vi "host run 2.vi"() -> ()   [LabVIEW 2012]
panel:
  out "Frame Rate":dbl
  out "Image":T1(plugin-control)
  in  "stop":bool
  out "Image 2":T1(plugin-control)
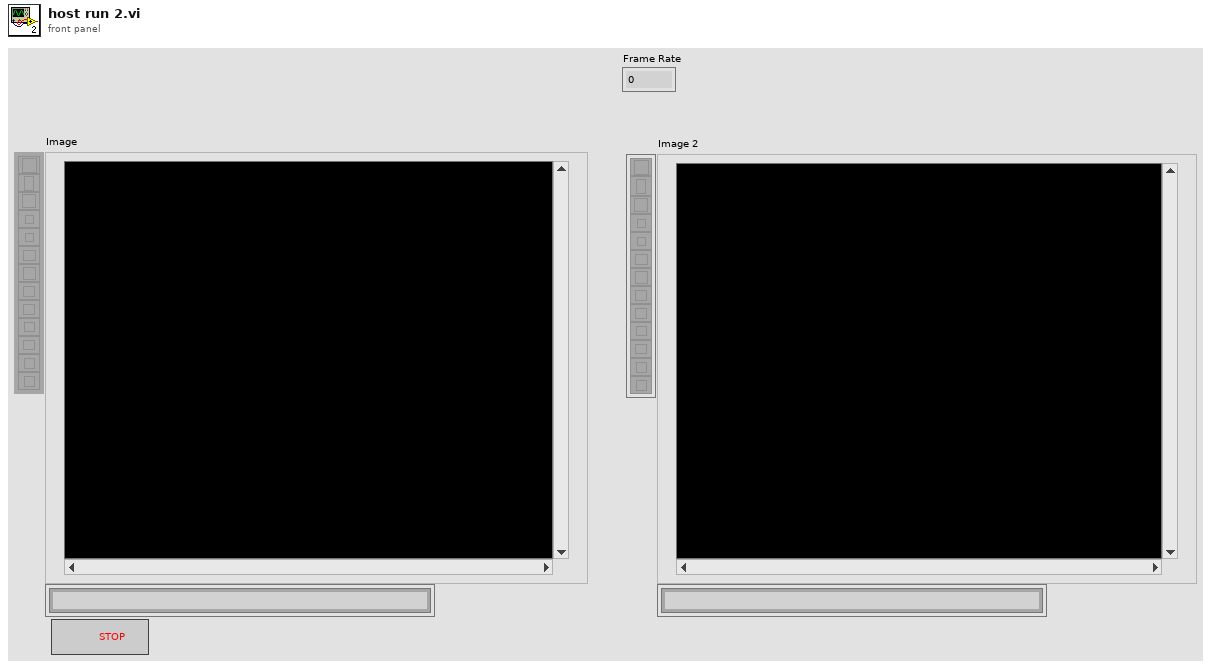
[diagram p1: front panel]
types:
  T1 = typedef "IMAQ Image.ctl" = refnum<image>
  T2 = cluster{"Global Rectangle":cluster{"x1Left":i32, "y1Top":i32, "x2Right":i32, "y2Bottom":i32}, "Centroid":cluster{"x":sgl, "y":sgl}, "Object Size":u32, "Score":dbl}[]
  T3 = cluster{"Shape Report (Shape Matching 1)[0]":cluster{"Global Rectangle":cluster{"x1Left":i32, "y1Top":i32, "x2Right":i32, "y2Bottom":i32}, "Centroid":cluster{"x":sgl, "y":sgl}, "Object Size":u32, "Score":dbl}, "Shape Report (Shape Matching 1)[1]":cluster{"Global Rectangle":cluster{"x1Left":i32, "y1Top":i32, "x2Right":i32, "y2Bottom":i32}, "Centroid":cluster{"x":sgl, "y":sgl}, "Object Size":u32, "Score":dbl}, "Shape Report (Shape Matching 1)[2]":cluster{"Global Rectangle":cluster{"x1Left":i32, "y1Top":i32, "x2Right":i32, "y2Bottom":i32}, "Centroid":cluster{"x":sgl, "y":sgl}, "Object Size":u32, "Score":dbl}, "Shape Report (Shape Matching 1)[3]":cluster{"Global Rectangle":cluster{"x1Left":i32, "y1Top":i32, "x2Right":i32, "y2Bottom":i32}, "Centroid":cluster{"x":sgl, "y":sgl}, "Object Size":u32, "Score":dbl}, "Shape Report (Shape Matching 1)[4]":cluster{"Global Rectangle":cluster{"x1Left":i32, "y1Top":i32, "x2Right":i32, "y2Bottom":i32}, "Centroid":cluster{"x":sgl, "y":sgl}, "Object Size":u32, "Score":dbl}, "Shape Report (Shape Matching 1)[5]":cluster{"Global Rectangle":cluster{"x1Left":i32, "y1Top":i32, "x2Right":i32, "y2Bottom":i32}, "Centroid":cluster{"x":sgl, "y":sgl}, "Object Size":u32, "Score":dbl}, "Shape Report (Shape Matching 1)[6]":cluster{"Global Rectangle":cluster{"x1Left":i32, "y1Top":i32, "x2Right":i32, "y2Bottom":i32}, "Centroid":cluster{"x":sgl, "y":sgl}, "Object Size":u32, "Score":dbl}, "Shape Report (Shape Matching 1)[7]":cluster{"Global Rectangle":cluster{"x1Left":i32, "y1Top":i32, "x2Right":i32, "y2Bottom":i32}, "Centroid":cluster{"x":sgl, "y":sgl}, "Object Size":u32, "Score":dbl}, "Shape Report (Shape Matching 1)[8]":cluster{"Global Rectangle":cluster{"x1Left":i32, "y1Top":i32, "x2Right":i32, "y2Bottom":i32}, "Centroid":cluster{"x":sgl, "y":sgl}, "Object Size":u32, "Score":dbl}}
  T4 = cluster{"x1Left":i32, "y1Top":i32, "x2Right":i32, "y2Bottom":i32}
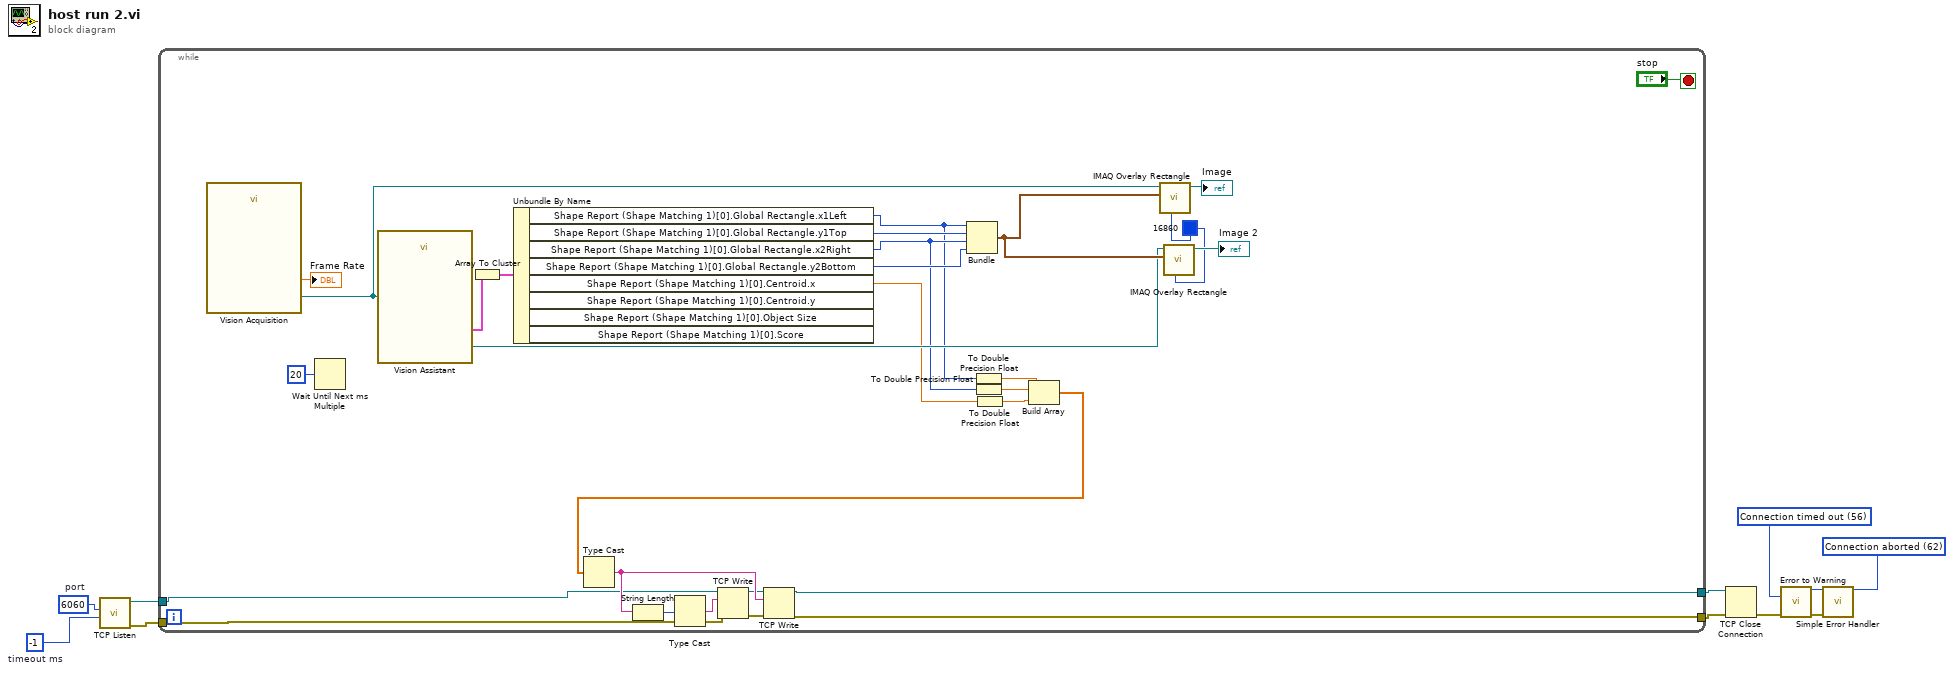
[diagram p0: block diagram]
diagram:
  w3 = 56 items=["No Error", "Argument Error", "Memory Full", "Out of Zone", "End of File", "File Already Open", "Generic File IO Error", "File Not Found", "File Permission Error", "Disk Full", "Duplicate Path", "Too Many Files Open", "Not Enabled", "Resource File Not Found", "Cannot Add Resource", "Resource Not Found", "Image Not Found", "Image Memory Error", "Pen Does Not Exist", "Config Bad Type", "Config Token Not Found", "Config Parse Error", "Config Memory Error", "Bad External Code Format", "Bad External Code Offset", "External Code Not Present", "Null Window", "Destroy Window Mixup", "Null Menu", "Print Aborted", "Bad Print Record", "Print Driver Error", "Windows Error During Print", "Memory Error During Print", "Print Dialog Error", "Generic Print Error", "Invalid Device Refnum", "Device Not Found", "Device Parameter Error", "Device Unit Error", "Can't Open Device", "Device Call Aborted", "Generic Error", "Cancelled By User", "Object ID Too Low", "Object ID Too High", "Object Not In Heap", "Unknown Heap", "Bad DefProc ID", "DefProc Not In Table", "Message Out Of Range", "Null Method", "Unknown Message", "Manager Call Not Supported", "Bad address", "Connection In progress", "Connection timed out", "Connection is already in progress", "Network attribute not supported", "Network error", "Address in use", "System out of memory", "Connection aborted", "Connection refused", "Connection is not connected", "Connection is already connected", "Connection closed", "Initialize error (interapplication manager)", "Bad occurrence", "Wait on unbound occurrence handler", "Occurrence queue overflow", "Bad path", "Semaphore not signaled", "Unrecognized type (interapplication manager)"] ("2nd Error to Convert")
  w4 = 62 items=["No Error", "Argument Error", "Memory Full", "Out of Zone", "End of File", "File Already Open", "Generic File IO Error", "File Not Found", "File Permission Error", "Disk Full", "Duplicate Path", "Too Many Files Open", "Not Enabled", "Resource File Not Found", "Cannot Add Resource", "Resource Not Found", "Image Not Found", "Image Memory Error", "Pen Does Not Exist", "Config Bad Type", "Config Token Not Found", "Config Parse Error", "Config Memory Error", "Bad External Code Format", "Bad External Code Offset", "External Code Not Present", "Null Window", "Destroy Window Mixup", "Null Menu", "Print Aborted", "Bad Print Record", "Print Driver Error", "Windows Error During Print", "Memory Error During Print", "Print Dialog Error", "Generic Print Error", "Invalid Device Refnum", "Device Not Found", "Device Parameter Error", "Device Unit Error", "Can't Open Device", "Device Call Aborted", "Generic Error", "Cancelled By User", "Object ID Too Low", "Object ID Too High", "Object Not In Heap", "Unknown Heap", "Bad DefProc ID", "DefProc Not In Table", "Message Out Of Range", "Null Method", "Unknown Message", "Manager Call Not Supported", "Bad address", "Connection In progress", "Connection timed out", "Connection is already in progress", "Network attribute not supported", "Network error", "Address in use", "System out of memory", "Connection aborted", "Connection refused", "Connection is not connected", "Connection is already connected", "Connection closed", "Initialize error (interapplication manager)", "Bad occurrence", "Wait on unbound occurrence handler", "Occurrence queue overflow", "Bad path", "Semaphore not signaled", "Unrecognized type (interapplication manager)"] ("1st Error to Convert")
  w9 = u16 6060  # port
  w10 = -1  # timeout ms
  n1 = call <vilib>:"TCP Listen.vi"("timeout ms (wait forever: -1)"=w10, "port"=w9) -> ("error out"=w7:errorcluster, "connection ID"=w8:refnum<k5>)  [unwired: 5 in, 3 out]
  n2 = while {
    tunnel: w8 -> [w24]
    tunnel: w7 -> [w25]
    tunnel: [w23] -> w1
    tunnel: [w22] -> w2
    stop <- "stop" stop-if-true
    w32 = u32 16860 ("Color")
    n3 = call "Vision Acquisition"() -> ("Image Out"=w21:T1, "Frame Rate"=→"Frame Rate":dbl)  [unwired: 24 in, 2 out]
    n4 = Wait Until Next ms Multiple(millisecond multiple=u32 20) -> ()  [unwired: 1 out]
    n5 = call "Vision Assistant"("Image In"=w21) -> ("Image Out"=w19:T1, "Shape Report (Shape Matching 1)"=w20:T2)  [unwired: 23 in, 2 out]
    n6 = Array To Cluster(array=w20) -> (cluster=w39:T3)
    n7 = Unbundle By Name(w39) -> ("Shape Report (Shape Matching 1)[0].Global Rectangle.x1Left"=w13:i32, "Shape Report (Shape Matching 1)[0].Global Rectangle.y1Top"=w37:i32, "Shape Report (Shape Matching 1)[0].Global Rectangle.x2Right"=w14:i32, "Shape Report (Shape Matching 1)[0].Global Rectangle.y2Bottom"=w36:i32, "Shape Report (Shape Matching 1)[0].Centroid.x"=w15:sgl)  [unwired: 3 out]
    n8 = Bundle("x1Left"=w13, "y1Top"=w37, "x2Right"=w14, "y2Bottom"=w36) -> (w33:T4)  [unwired: 1 in]
    n9 = To Double Precision Float(number=w13) -> (double precision float=w18:dbl)
    n10 = To Double Precision Float(number=w14) -> (double precision float=w17:dbl)
    n11 = To Double Precision Float(number=w15) -> (double precision float=w16:dbl)
    n12 = Build Array(w18, w17, w16) -> (w12:dbl[])
    n13 = Type Cast(x=w12) -> (*(type *) &x=w30:string)  [unwired: 1 in]
    n14 = String Length(string=w30) -> (length=w28:i32)
    n15 = Type Cast(x=w28) -> (*(type *) &x=w29:string)  [unwired: 1 in]
    n16 = TCP Write(connection ID=w24, data in=w29, error in (no error)=w25) -> (connection ID out=w26:refnum<k5>, error out=w27:errorcluster)  [unwired: 1 in, 1 out]
    n17 = TCP Write(connection ID=w26, data in=w30, error in (no error)=w27) -> (connection ID out=w23:refnum<k5>, error out=w22:errorcluster)  [unwired: 1 in, 1 out]
    n18 = call "IMAQ Overlay Rectangle"("Color"=w32, "Rectangle"=w33, "Image"=w21) -> ("Image Out"=→"Image":T1)  [unwired: 7 in, 1 out]
    n19 = call "IMAQ Overlay Rectangle"("Color"=w32, "Rectangle"=w33, "Image"=w19) -> ("Image Out"=→"Image 2":T1)  [unwired: 7 in, 1 out]
  }
  n20 = TCP Close Connection(connection ID=w1, error in (no error)=w2) -> (error out=w6:errorcluster)  [unwired: 1 in, 1 out]
  n21 = call <vilib>:"Error to Warning.vi"("1st Error to Convert"=w4, "2nd Error to Convert"=w3, "error in"=w6) -> ("warning out"=w5:errorcluster)  [unwired: 12 in]
  n22 = call <vilib>:"Simple Error Handler.vi"("error in (no error)"=w5) -> ()  [unwired: 4 in, 5 out]
